vi "gyro -- async pll engine.vi"(11 "pll event pair":T8) -> ()   [LabVIEW 2020]
uses:
  PID action.ctl
  pll parameters.ctl
  PID - mode.ctl
  lorentzian.ctl
  circle corners.ctl
  pll talkback data type.ctl
  server talk-to-back pair.ctl
  server talkback message type.ctl
  server talkto message type.ctl
  pid -- parameters.ctl
  agregator -- action.ctl
  interpolation state - real.ctl
  data source action.ctl
  four-corner circle transformation.ctl
  publisher action.ctl
  linear interpolation - real.vi
  Q -- check range -- i -- real.vi
  linear interpolation iiii- complex.vi
  <vilib>/Analysis/baseanly.llb/A x B.vi
  <vilib>/Analysis/baseanly.llb/Complex A x B.vi
  line -- complex.vi
  Q -- check range -- i -- integer.vi
  Q - not nan -- real.vi
  Q - not nan -- integer.vi
  <vilib>/Analysis/Matrix/Numeric/Conversions/Array To Matrix.vi
  <vilib>/Analysis/Matrix/Numeric/Conversions/Array To Matrix - RA2.vi
  <vilib>/Analysis/baseanly.llb/Inverse Matrix.vi
  <vilib>/Analysis/baseanly.llb/Real Inverse Matrix.vi
panel:
  in  "main":enum32{"Page 1", "Page 2", "Page 3"}(tab)
  in  "pll parameters":T1={"PID mode"=enum."normal", "plot hist time (sec)"=1.0, "dt (sec)"=0.0005, "visc hist time (sec)"=2.0, "time int ave time (sec)"=0.3, "PLL limits (Hz)"=5000.0} {"PLL limits (Hz)" format="%#.2f"; "time int ave time (sec)" format="%#_10f"; "visc hist time (sec)" format="%#_10f"; "dt (sec)" format="%#_10f"; "plot hist time (sec)" format="%#_10f"}
  in  "PID parameters :{}[];'":T3={"I (sec)"=0.004634123928756344, "P (sec)"=0.008980860327047186} {"P (sec)" scale=0.01..10.0; "I (sec)" scale=0.01..10.0}
  out "results":T4={"freq (Hz)"=6.94529631676717e-310, "gamma (Hz)"=inf, "Voltage (V)"=1e-323+8e-323i, "overlimit ?"=FALSE} {"Voltage (V)" format="%#.4f"; "gamma (Hz)" format="%#.4f"; "freq (Hz)" format="%#.11f"}
  out "PLL is ON ?":bool
  out "owl mode !":bool
  in  "Do reset frequency -- PID action":T5=enum."reset frequency"
  in  "Do reset frequency source":dbl=15.0 format="%#_10f"
  out "zi freq temporary":dbl=40015.59220124337 format="%#.2f"
  out "DO reset freq !":bool
  in  "lorentzian":T6={"A (VHz)"=1.0, "f (Hz)"=1000.0, "G (Hz)"=3.0, "phi(rad)"=0.0, "Q"=300.0, "Norm  Ampl"=nan, "bg (V)"=0.0+0.0i, "4corners"={"z (-pi/2)"=9.277908004825974e-07+0.0007240755403629966i, "z(inf)"=2.6527949823343002e-05+0.0007477540585896028i, "z (pi/2)"=2.8494315967368497e-06+0.0007733542176124632i, "z center"=1.8886111986097237e-06+0.0007487148789877299i, "z(0)"=-2.2750727426123552e-05+0.000749675699385857i, "radius"=2.4658065287076567e-05}} {"bg (V)" format="%#9_9f"; "Q" format="%#9_9f"; "phi(rad)" format="%#9_9f"; "G (Hz)" format="%#9_9f"; "f (Hz)" format="%#9_9f"}
  out "Numeric":i32=324
  out "Stoped?":bool=TRUE
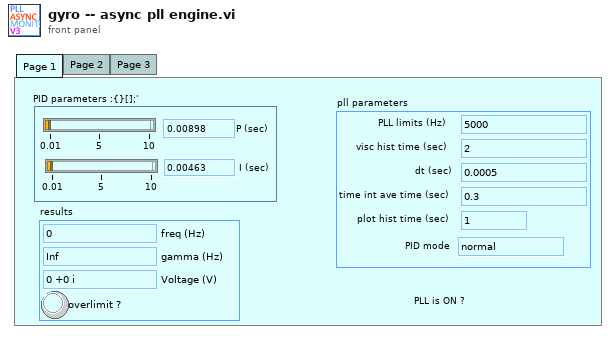
[diagram p1: front panel]
types:
  T1 = typedef "pll parameters.ctl" = cluster{"PID mode":T2, "plot hist time (sec)":dbl, "dt (sec)":dbl, "visc hist time (sec)":dbl, "time int ave time (sec)":dbl, "PLL limits (Hz)":dbl}
  T2 = typedef "PID - mode.ctl" = enum16{"normal", "heat"}
  T3 = typedef "pid -- parameters.ctl" = cluster{"I (sec)":dbl, "P (sec)":dbl}
  T4 = typedef "pll talkback data type.ctl" = cluster{"freq (Hz)":dbl, "gamma (Hz)":dbl, "Voltage (V)":cdb, "overlimit ?":bool}
  T5 = typedef "PID action.ctl" = enum16{"append", "empty!", "reset frequency", "reset from num", "overlimit"}
  T6 = typedef "lorentzian.ctl" = cluster{"A (VHz)":dbl, "f (Hz)":dbl, "G (Hz)":dbl, "phi(rad)":dbl, "Q":dbl, "Norm  Ampl":dbl, "bg (V)":cdb, "4corners":T7}
  T7 = typedef "circle corners.ctl" = cluster{"z (-pi/2)":cdb, "z(inf)":cdb, "z (pi/2)":cdb, "z center":cdb, "z(0)":cdb, "radius":dbl}
  T8 = typedef "server talk-to-back pair.ctl" = cluster{"talkback event":refnum<user-event>, "talkto event":refnum<user-event>}
  T9 = typedef "interpolation state - real.ctl" = cluster{"requested size":i32, "Array":dbl[], "actual number of elements":i32}
  T10 = typedef "agregator -- action.ctl" = enum16{"append", "interpolate", "empty!", "force", "init", "scale", "read last"}
  T11 = typedef "server talkback message type.ctl" = cluster{"message":enum16{"new", "void"}}
  T12 = typedef "publisher action.ctl" = enum16{"set", "get", "init", "check"}
  T13 = typedef "data source action.ctl" = enum16{"set", "get", "init", "set-and-get", "init source"}
  T14 = typedef "four-corner circle transformation.ctl" = enum16{"z(c) z(inf)", "z(c) z(zero)", "fix phase", "calculate lorentzian", "z(0) z(+-pi/2)", "shift to zcenter", "to  canonical", "get canonical phase", "get4corners", "update lorentzian -- from z0", "fake gamma normal", "fake gamma heat", "calculate complex slope"}
  T15 = typedef "PLL data source.ctl" = enum16{"meta", "MFLI", "SRS865A", "arydh"}
  T16 = typedef "interpolation state - complex.ctl" = cluster{"requested size":i32, "Array":cdb[], "actual number of elements":i32}
  T17 = typedef "eventvkey.ctl" = enum16{"ASCII", "Enter", "Return", "Shift", "Ctrl", "Alt", "Cmd", "Opt", "Caps", "NumLock", "Clear", "Break", "Up", "Down", "Left", "Right", "Insert", "Delete", "Home", "End", "PageUp", "PageDown", "Escape", "Help", "Pause", "ScrollLock", "F1", "F2", "F3", "F4", "F5", "F6", "F7", "F8", "F9", "F10", "F11", "F12", "F13", "F14", "F15", "F16", "F17", "F18", "F19", "F20", "F21", "F22", "F23", "F24", "Play", "VolumeUp", "VolumeDown", "Mute", "Two Byte Char"}
  T18 = enum16{"stop", "start", "update pars", "update request", "new", "launch", "exit", "get", "reset", "pause", "unpause"}
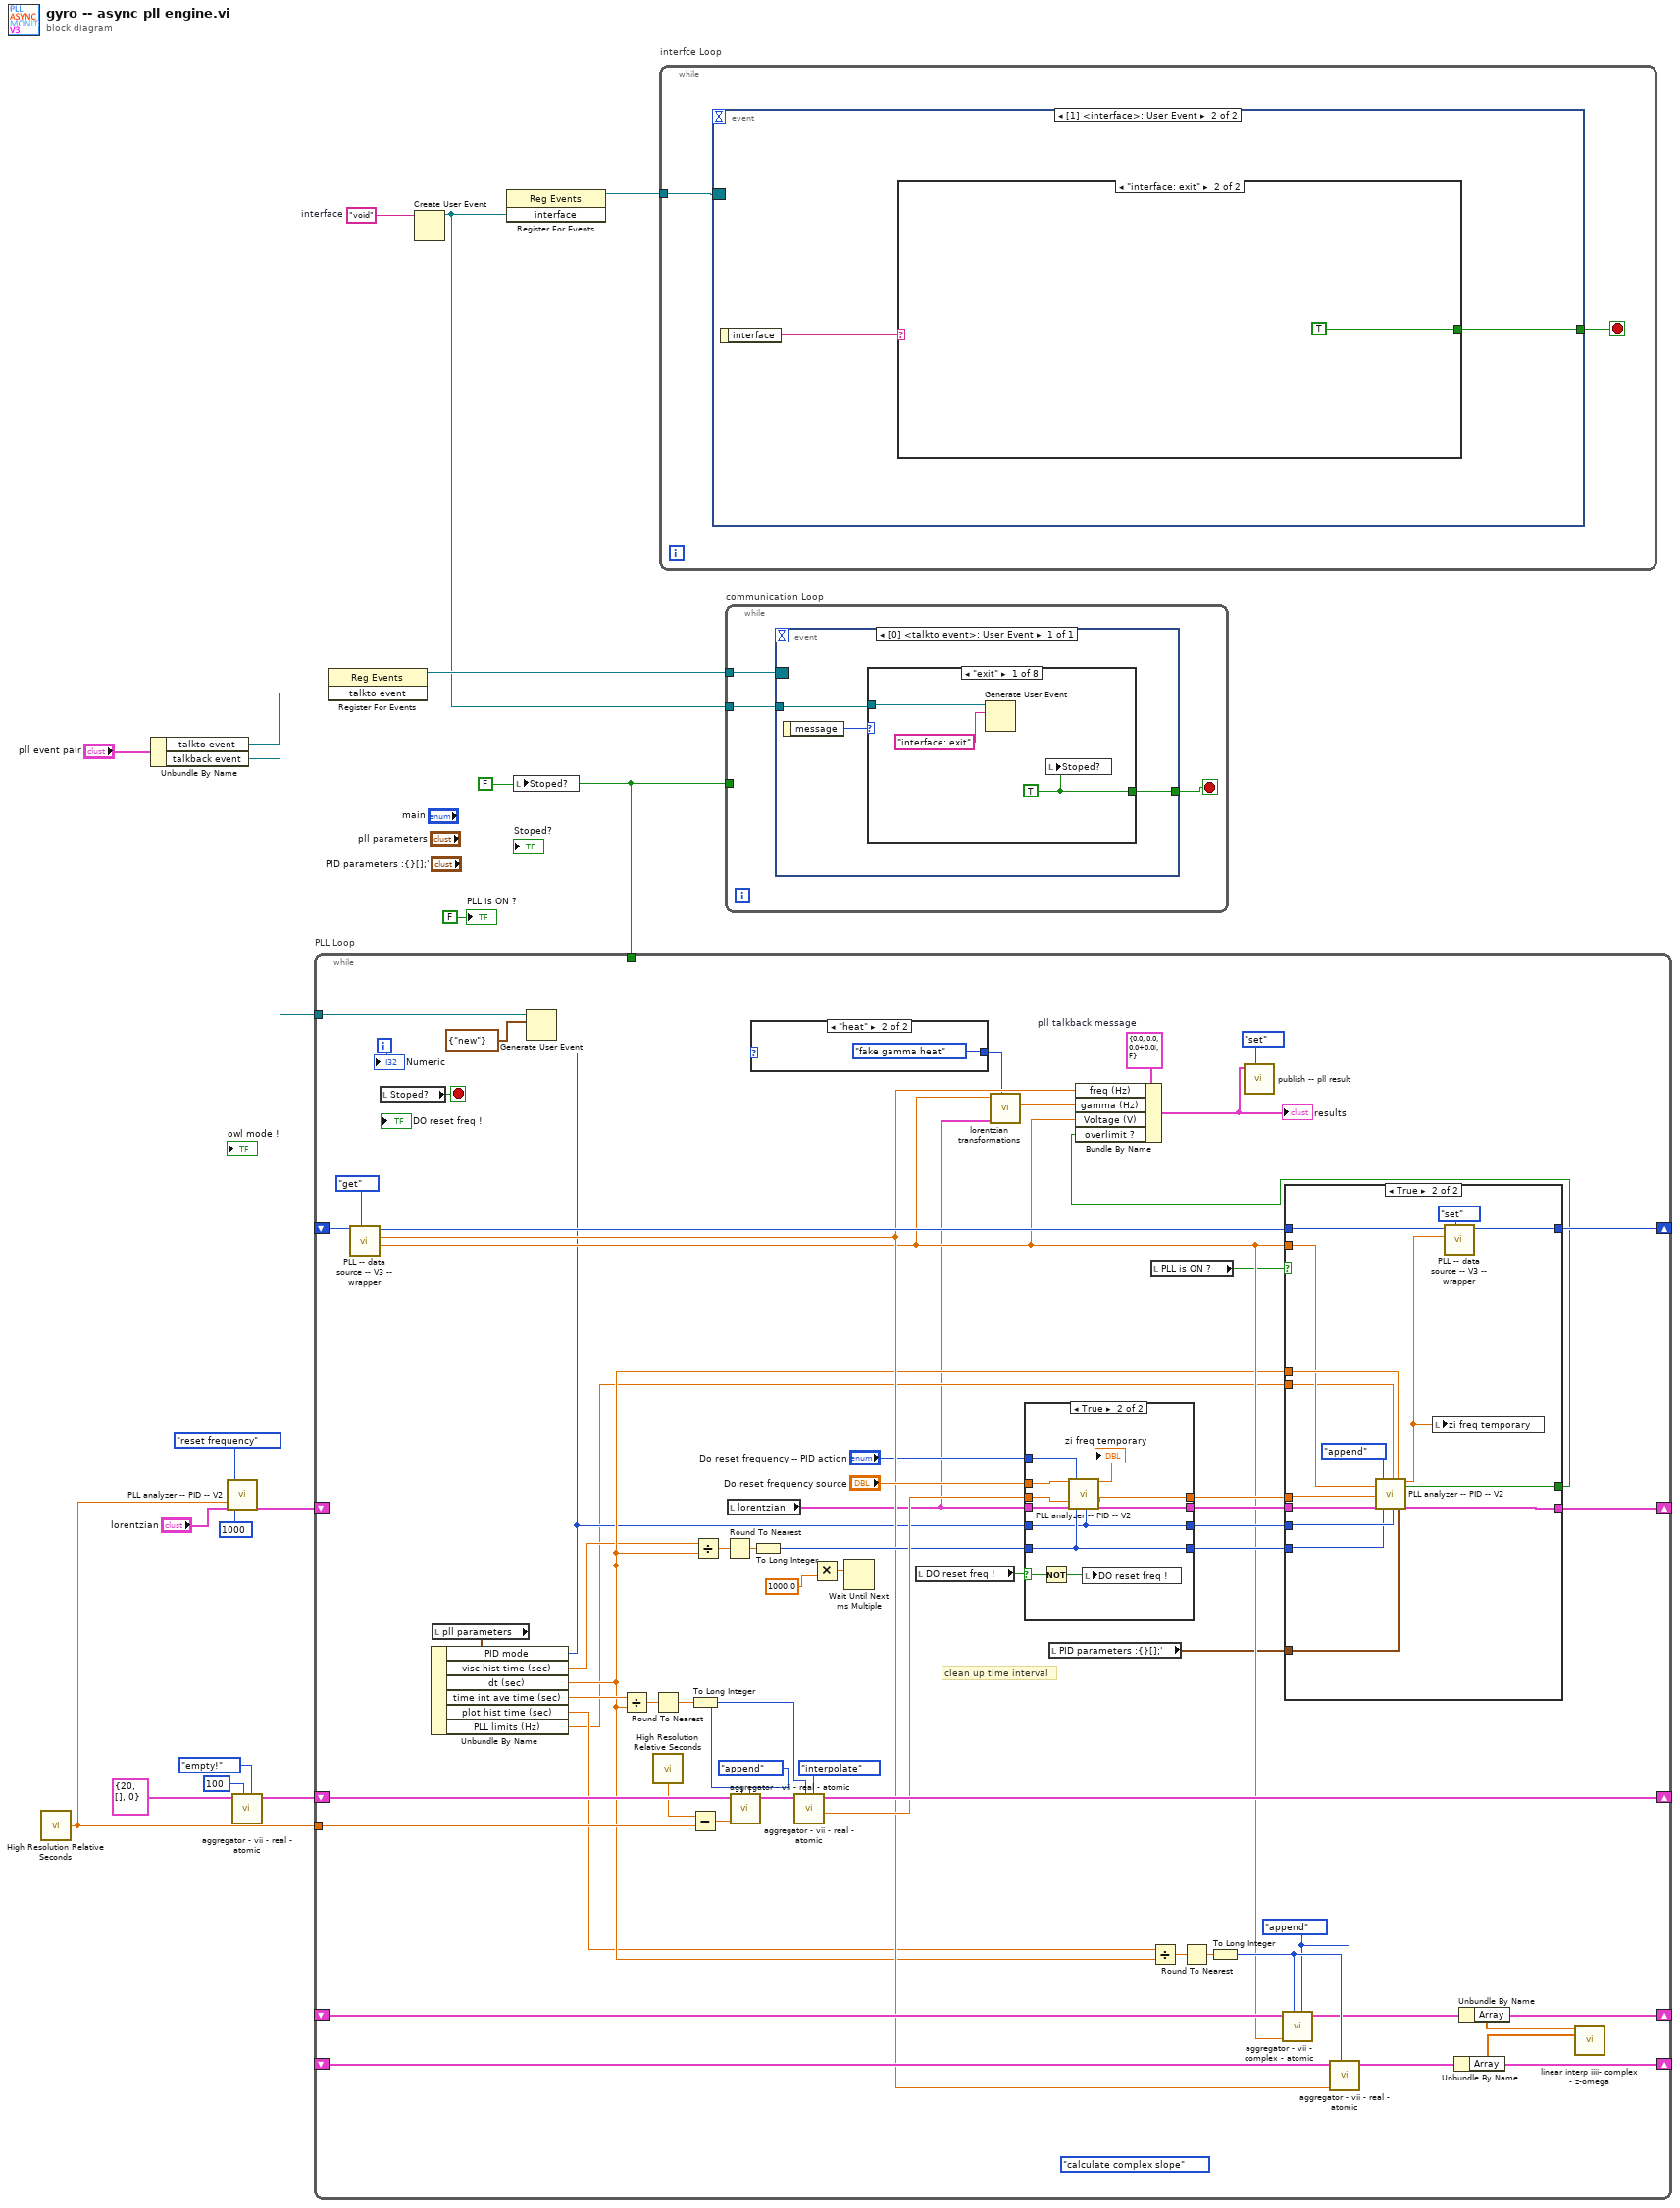
[diagram p0: block diagram]
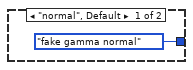
[diagram p2: hidden frame]
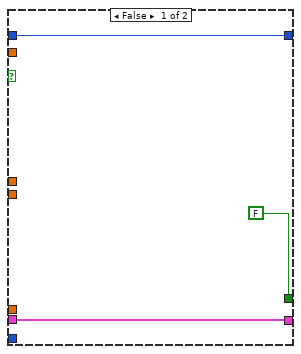
[diagram p3: hidden frame]
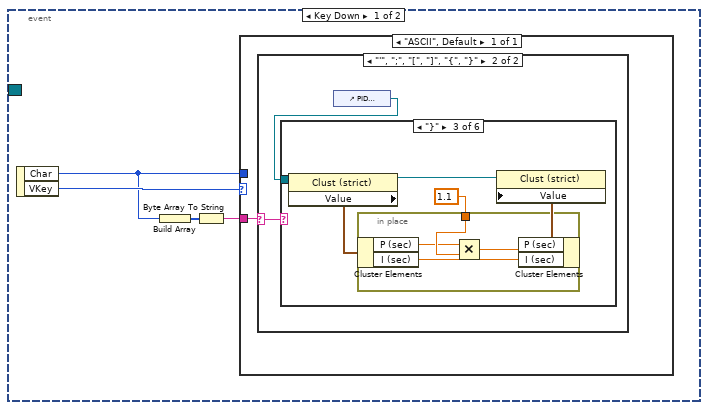
[diagram p5: hidden frame]
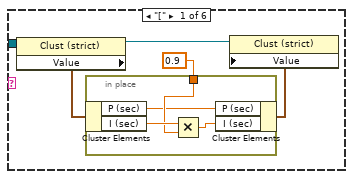
[diagram p7: hidden frame]
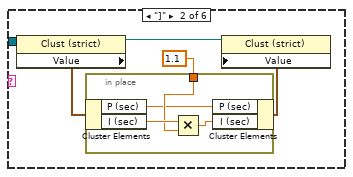
[diagram p8: hidden frame]
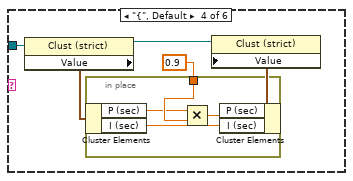
[diagram p9: hidden frame]
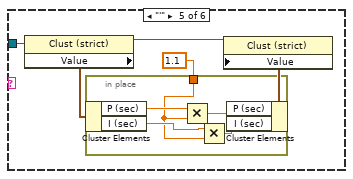
[diagram p10: hidden frame]
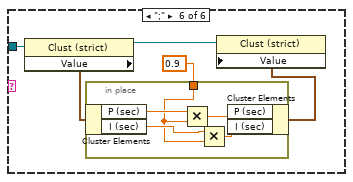
[diagram p11: hidden frame]
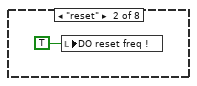
[diagram p13: hidden frame]
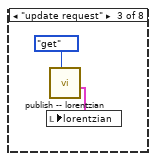
[diagram p14: hidden frame]
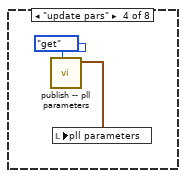
[diagram p15: hidden frame]
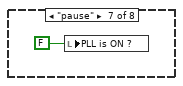
[diagram p18: hidden frame]
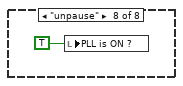
[diagram p19: hidden frame]
diagram:
  w3 = "void"  # interface
  w4 = FALSE ("Stop")
  n1 = call <vilib>:"High Resolution Relative Seconds.vi"() -> ("relative seconds"=w6:dbl)
  n2 = Unbundle By Name("pll event pair") -> ("talkto event"=w14:refnum<user-event>, "talkback event"=w15:refnum<user-event>)
  n3 = call "PLL analyzer -- PID -- V2.vi"("time in (sec)"=w6, "lorentzian IN"="lorentzian", "PID action"=PID_action."reset frequency", "requested size"=1000) -> ("lorentzian  OUT"=w9:T6)  [unwired: 12 in, 3 out]
  n4 = call "aggregator - vii - real - atomic.vi"("aggregator action"=agregator_--_action."empty!", "requested size"=100, "state IN"=T9 {"requested size"=20, "Array"=[], "actual number of elements"=0}) -> ("state OUT"=w12:T9)  [unwired: 5 in, 3 out]
  n5 = while "PLL Loop" {
    tunnel: w6 -> [w79]
    shift-right: [w77] -> _
    shift-left: w9 -> [_]
    shift-right: [w45] -> _
    shift-left: _ -> [w76]
    shift-right: [w74] -> _
    shift-left: _ -> [w75]
    shift-right: [w69] -> _
    shift-left: w12 -> [w72]
    shift-right: [w64] -> _
    shift-left: _ -> [w60]
    tunnel: w15 -> [w22]
    tunnel: w4 -> [_]
    i -> [w19]
    stop <- w25 stop-if-true
    w37 = T4 {"freq (Hz)"=0.0, "gamma (Hz)"=0.0, "Voltage (V)"=0.0+0.0i, "overlimit ?"=FALSE}  # pll talkback message
    (unwired) four-corner_circle_transformation."calculate complex slope" ("4 corner circle transformation")
    w20 = agregator_--_action."append" ("aggregator action")
    # "clean up time interval"
    n6 = call "PLL -- data source -- V3 -- wrapper.vi"("data source action"=data_source_action."get", "PLL data source"=w60) -> ("z out (V)"=w40:cdb, "Freq out (Hz)"=w44:dbl, "PLL data source OUT"=w62:T15)  [unwired: 7 in]
    n7 = local read "Stoped?"() -> (w25:bool)
    n8 = local read "pll parameters"() -> (w32:T1)
    n9 = Unbundle By Name(w32) -> ("PID mode"=w33:T2, "visc hist time (sec)"=w34:dbl, "dt (sec)"=w35:dbl, "time int ave time (sec)"=w36:dbl, "plot hist time (sec)"=w31:dbl, "PLL limits (Hz)"=w29:dbl)
    n10 = Generate User Event(user event=w22, event data cluster=T11 {"message"=enum."new"} ("event data")) -> ()  [unwired: 2 in, 2 out]
    n11 = Divide(x=w36, y=w35) -> (x/y=w53:dbl)
    n12 = Round To Nearest(number=w53) -> (nearest integer value=w52:dbl)
    n13 = call <vilib>:"High Resolution Relative Seconds.vi"() -> ("relative seconds"=w63:dbl)
    n14 = To Long Integer(number=w52) -> (32bit integer=w51:i32)
    n15 = Subtract(x=w63, y=w79) -> (x-y=w71:dbl)
    n16 = Divide(x=w34, y=w35) -> (x/y=w56:dbl)
    n17 = Round To Nearest(number=w56) -> (nearest integer value=w55:dbl)
    n18 = local read "lorentzian"() -> (w26:T6)
    n19 = call "aggregator - vii - real - atomic.vi"("aggregator action"=agregator_--_action."append", "requested size"=w51, "number"=w71, "state IN"=w72) -> ("state OUT"=w70:T9)  [unwired: 4 in, 3 out]
    n20 = case shown="\"heat\"" w33 {
      tunnel: [four-corner_circle_transformation."fake gamma normal" ("4 corner circle transformation") four-corner_circle_transformation."fake gamma heat" ("4 corner circle transformation")] -> w42
      frame "normal", Default {
      }
      frame "heat" {
      }
    }
    n21 = To Long Integer(number=w55) -> (32bit integer=w54:i32)
    n22 = call "aggregator - vii - real - atomic.vi"("aggregator action"=agregator_--_action."interpolate", "requested size"=w51, "state IN"=w70) -> ("interp average"=w58:dbl, "state OUT"=w69:T9)  [unwired: 5 in, 2 out]
    n23 = Multiply(x=w35, y=1000.0) -> (x*y=w67:dbl)
    n24 = Wait Until Next ms Multiple(millisecond multiple=w67) -> ()  [unwired: 1 out]
    n25 = local read "DO reset freq !"() -> (w66:bool)
    n26 = call "lorentzian transformations.vi"("4 corner circle transformation"=w42, "lorentzian in"=w26, "voltage in"=w40) -> ("gamma OUT"=w41:dbl)  [unwired: 5 in, 3 out]
    n27 = case shown="True" w66 {
      selector: w66 -> [_ w112]
      tunnel: w26 -> [w103 w114]
      tunnel: [w103 w113] -> w65
      tunnel: w54 -> [w102 w109]
      tunnel: [w102 w109] -> w59
      tunnel: w58 -> [w101 w108]
      tunnel: "Do reset frequency -- PID action" -> [_ w107]
      tunnel: "Do reset frequency source" -> [_ w106]
      tunnel: [w101 w105] -> w50
      tunnel: w33 -> [w100 w104]
      tunnel: [w100 w104] -> w46
      frame False {
      }
      frame True {
        n28 = Not(x=w112) -> (.not. x?=w111:bool)
        n29 = call "PLL analyzer -- PID -- V2.vi"("frequency IN (Hz)"=w106, "time in (sec)"=w108, "lorentzian IN"=w114, "PID action"=w107, "requested size"=w109, "PID mode"=w104) -> ("frequency OUT (Hz)"=→"zi freq temporary":dbl, "time out (sec)"=w105:dbl, "lorentzian  OUT"=w113:T6)  [unwired: 10 in, 1 out]
        n30 = local write "DO reset freq !"(w111) -> ()
      }
    }
    n31 = local read "PID parameters :{}[];'"() -> (w23:T3)
    n32 = Divide(x=w31, y=w35) -> (x/y=w49:dbl)
    n33 = local read "PLL is ON ?"() -> (w24:bool)
    n34 = Round To Nearest(number=w49) -> (nearest integer value=w48:dbl)
    n35 = To Long Integer(number=w48) -> (32bit integer=w47:i32)
    n36 = call "aggregator - vii - complex - atomic.vi"("aggregator action"=w20, "requested size"=w47, "number"=w40, "state IN"=w76) -> ("state OUT"=w45:T16)  [unwired: 4 in, 3 out]
    n37 = case shown="True" w24 {
      tunnel: [w84 w99] -> w77
      tunnel: w59 -> [_ w90]
      tunnel: w40 -> [_ w88]
      tunnel: w50 -> [_ w94]
      tunnel: w65 -> [w84 w91]
      tunnel: [w83 w97] -> w64
      tunnel: w62 -> [w83 w95]
      tunnel: w35 -> [_ w93]
      tunnel: w46 -> [_ w92]
      tunnel: w23 -> [_ w87]
      tunnel: [FALSE w86] -> w30
      tunnel: w29 -> [_ w85]
      frame False {
      }
      frame True {
        n38 = call "PLL analyzer -- PID -- V2.vi"("voltage IN (V)"=w88, "time in (sec)"=w94, "lorentzian IN"=w91, "PID action"=PID_action."append", "requested size"=w90, "PLL limits (Hz)"=w85, "PID mode"=w92, "dt (sec)"=w93, "PID parameters"=w87) -> ("frequency OUT (Hz)"=w89:dbl, "overlimit ?"=w86:bool, "lorentzian  OUT"=w99:T6)  [unwired: 7 in, 1 out]
        n39 = local write "zi freq temporary"(w89) -> ()
        n40 = call "PLL -- data source -- V3 -- wrapper.vi"("data source action"=data_source_action."set", "Freq in (Hz)"=w89, "PLL data source"=w95) -> ("PLL data source OUT"=w97:T15)  [unwired: 6 in, 2 out]
      }
    }
    n41 = Bundle By Name(cluster=w37, "freq (Hz)"=w44, "gamma (Hz)"=w41, "Voltage (V)"=w40, "overlimit ?"=w30) -> (w28:T4)
    "results" <- w28
    n42 = call "publish -- pll result.vi"("publisher action"=publisher_action."set", "pll result IN"=w28) -> ()  [unwired: 9 in, 1 out]
    n43 = call "aggregator - vii - real - atomic.vi"("aggregator action"=w20, "requested size"=w47, "number"=w44, "state IN"=w75) -> ("state OUT"=w74:T9)  [unwired: 4 in, 3 out]
    n44 = Unbundle By Name(w74) -> ("Array"=w38:dbl[])
    n45 = Unbundle By Name(w45) -> ("Array"=w39:cdb[])
    n46 = call "linear interp iiii- complex - z-omega.vi"("z"=w39, "omega"=w38) -> ()  [unwired: 5 in, 9 out]
    "Numeric" <- w19
  }
  n47 = register-events(w14) -> (reference out=w18:refnum<event-registration>)  [unwired: 2 in, 1 out]
  n48 = Create User Event(user event datatype=w3) -> (user event=w1:refnum<user-event>)  [unwired: 1 in, 1 out]
  n49 = register-events(w1) -> (reference out=w2:refnum<event-registration>)  [unwired: 2 in, 1 out]
  n50 = local write "Stoped?"(w4) -> ()
  n51 = while "interfce Loop" {
    tunnel: w2 -> [w116]
    stop <- w115 stop-if-true
    n52 = event shown="[1] <interface>: User Event" {
      selector: w116 -> [_ _]
      dyn-events: _ -> [_ _]
      timeout: _ -> [_ _]
      tunnel: [_ w180] -> w115
      event Key Down {
        n53 = event-data() -> ("Char"=w118:i16, "VKey"=w120:T17)  [unwired: 1 in]
        n54 = Build Array(w118) -> (w119:i16[])
        n55 = Byte Array To String(unsigned byte array=w119) -> (string=w117:string)
        n56 = case shown="\"ASCII\", Default" w120 {
          tunnel: w118 -> [_]
          tunnel: w117 -> [w121]
          frame "ASCII", Default {
            n57 = case shown="\"'\", \";\", \"[\", \"]\", \"{\", \"}\"" w121 {
              selector: w121 -> [_ w123]
              frame "0", Default {
              }
              frame "'", ";", "[", "]", "{", "}" {
                n58 = control-ref of="PID parameters :{}[];'"() -> (w122:refnum<vi>)
                n59 = case shown="\"}\"" w123 {
                  tunnel: w122 -> [w128 w137 w146 w155 w164 w174]
                  frame "[" {
                    n60 = property class="Clust (strict)"(reference=w128) -> (reference out=w127:refnum<vi>, "Value"=w126:T3)  [unwired: 1 in, 1 out]
                    n61 = in-place {
                      in-place-border: 0.9 -> [w131]
                      n62 = in-place-cluster #1(w126) -> ("P (sec)"=w129:dbl, "I (sec)"=w132:dbl)
                      n63 = Multiply(x=w132, y=w131) -> (x*y=w130:dbl)
                      n64 = in-place-cluster #1("P (sec)"=w129, "I (sec)"=w130) -> (w125:T3)
                    }
                    n65 = property class="Clust (strict)"(reference=w127, "Value"=w125) -> ()  [unwired: 1 in, 2 out]
                  }
                  frame "]" {
                    n66 = property class="Clust (strict)"(reference=w137) -> (reference out=w136:refnum<vi>, "Value"=w135:T3)  [unwired: 1 in, 1 out]
                    n67 = in-place {
                      in-place-border: 1.1 -> [w140]
                      n68 = in-place-cluster #2(w135) -> ("P (sec)"=w138:dbl, "I (sec)"=w141:dbl)
                      n69 = Multiply(x=w141, y=w140) -> (x*y=w139:dbl)
                      n70 = in-place-cluster #2("P (sec)"=w138, "I (sec)"=w139) -> (w134:T3)
                    }
                    n71 = property class="Clust (strict)"(reference=w136, "Value"=w134) -> ()  [unwired: 1 in, 2 out]
                  }
                  frame "}" {
                    n72 = property class="Clust (strict)"(reference=w146) -> (reference out=w145:refnum<vi>, "Value"=w144:T3)  [unwired: 1 in, 1 out]
                    n73 = in-place {
                      in-place-border: 1.1 -> [w150]
                      n74 = in-place-cluster #3(w144) -> ("P (sec)"=w149:dbl, "I (sec)"=w147:dbl)
                      n75 = Multiply(x=w149, y=w150) -> (x*y=w148:dbl)
                      n76 = in-place-cluster #3("P (sec)"=w148, "I (sec)"=w147) -> (w143:T3)
                    }
                    n77 = property class="Clust (strict)"(reference=w145, "Value"=w143) -> ()  [unwired: 1 in, 2 out]
                  }
                  frame "{", Default {
                    n78 = property class="Clust (strict)"(reference=w155) -> (reference out=w154:refnum<vi>, "Value"=w153:T3)  [unwired: 1 in, 1 out]
                    n79 = in-place {
                      in-place-border: 0.9 -> [w159]
                      n80 = in-place-cluster #4(w153) -> ("P (sec)"=w158:dbl, "I (sec)"=w156:dbl)
                      n81 = Multiply(x=w158, y=w159) -> (x*y=w157:dbl)
                      n82 = in-place-cluster #4("P (sec)"=w157, "I (sec)"=w156) -> (w152:T3)
                    }
                    n83 = property class="Clust (strict)"(reference=w154, "Value"=w152) -> ()  [unwired: 1 in, 2 out]
                  }
                  frame "'" {
                    n84 = property class="Clust (strict)"(reference=w164) -> (reference out=w163:refnum<vi>, "Value"=w162:T3)  [unwired: 1 in, 1 out]
                    n85 = in-place {
                      in-place-border: 1.1 -> [w165]
                      n86 = in-place-cluster #5(w162) -> ("P (sec)"=w169:dbl, "I (sec)"=w167:dbl)
                      n87 = Multiply(x=w169, y=w165) -> (x*y=w168:dbl)
                      n88 = Multiply(x=w167, y=w165) -> (x*y=w166:dbl)
                      n89 = in-place-cluster #5("P (sec)"=w168, "I (sec)"=w166) -> (w161:T3)
                    }
                    n90 = property class="Clust (strict)"(reference=w163, "Value"=w161) -> ()  [unwired: 1 in, 2 out]
                  }
                  frame ";" {
                    n91 = property class="Clust (strict)"(reference=w174) -> (reference out=w173:refnum<vi>, "Value"=w172:T3)  [unwired: 1 in, 1 out]
                    n92 = in-place {
                      in-place-border: 0.9 -> [w175]
                      n93 = in-place-cluster #6(w172) -> ("P (sec)"=w179:dbl, "I (sec)"=w177:dbl)
                      n94 = Multiply(x=w179, y=w175) -> (x*y=w178:dbl)
                      n95 = Multiply(x=w177, y=w175) -> (x*y=w176:dbl)
                      n96 = in-place-cluster #6("P (sec)"=w178, "I (sec)"=w176) -> (w171:T3)
                    }
                    n97 = property class="Clust (strict)"(reference=w173, "Value"=w171) -> ()  [unwired: 1 in, 2 out]
                  }
                }
              }
            }
          }
        }
      }
      event User Event {
        n98 = event-data() -> ("interface"=w181:string)  [unwired: 1 in]
        n99 = case shown="\"interface: exit\"" w181 {
          tunnel: [_ TRUE] -> w180
          frame "False", Default {
          }
          frame "interface: exit" {
          }
        }
      }
    }
  }
  n100 = while "communication Loop" {
    tunnel: w18 -> [w185]
    tunnel: w4 -> [_]
    tunnel: w1 -> [w183]
    stop <- w184 stop-if-true
    n101 = event shown="[0] <talkto event>: User Event" {
      selector: w185 -> [_]
      dyn-events: _ -> [_]
      timeout: _ -> [_]
      tunnel: [w187] -> w184
      tunnel: w183 -> [w186]
      event User Event {
        n102 = event-data() -> ("message"=w188:T18)  [unwired: 1 in]
        n103 = case shown="\"exit\"" w188 {
          tunnel: [w191 _ _ _ _ _ _ _] -> w187
          tunnel: w186 -> [w190 _ _ _ _ _ _ _]
          frame "exit" {
            w191 = TRUE
            n104 = Generate User Event(user event=w190, event data cluster="interface: exit" ("event data")) -> ()  [unwired: 2 in, 2 out]
            n105 = local write "Stoped?"(w191) -> ()
          }
          frame "reset" {
            n106 = local write "DO reset freq !"(TRUE) -> ()
          }
          frame "update request" {
            n107 = call "publish -- lorentzian.vi"("publisher action"=publisher_action."get") -> ("lorentzian OUT"=w193:T6)  [unwired: 10 in]
            n108 = local write "lorentzian"(w193) -> ()
          }
          frame "update pars" {
            n109 = call "publish -- pll parameters.vi"("publisher action"=publisher_action."get") -> ("pll parameters OUT"=w195:T1)  [unwired: 10 in]
            n110 = local write "pll parameters"(w195) -> ()
          }
          frame "start", Default {
          }
          frame "stop" {
          }
          frame "pause" {
            n111 = local write "PLL is ON ?"(FALSE ("Stoped?")) -> ()
          }
          frame "unpause" {
            n112 = local write "PLL is ON ?"(TRUE ("Stoped?")) -> ()
          }
        }
      }
    }
  }
  "PLL is ON ?" <- FALSE ("unpaused?")
